vi "OxyChip Calibration Prompt.vi"(11 "Measurement Information In":T1={"Comments"="", "Directory Input"="", "Data file path"=path "C:/Data/EPR Data", "Scripting File"=path "C:/Data/Configuration Script.csv", "Save Data"=FALSE, "Tooth size (d11) [mm]"=0.0, "Tooth size (d12) [mm]"=0.0, "Tooth size (d21) [mm]"=0.0, "Tooth size (d22) [mm]"=0.0, "Dose of Tooth [Gy]"=0.0, "Safe Shutdown?"=FALSE, "Gases Available"=[], "Database Username"="", "Database Password"="", "Database Login URL"="", "Database Upload URL"="", "Database Success URL"="", "Database XML URL"="", "Database Resonator URL"="", "Session Number"=0, "Set #"=0, "Resonator Operator"="", "Session Type"="", "Tooth/Sample ID"="", "Volunteer ID"="", "Computer Operator"="", "Volunteer Type"="", "Site/Tooth Selection (T8,T9)"="", "Resonator"="", "Measurement Site"="", "Non-standard session?"=FALSE, "EPR DAQ Version"="", "Session Path"=path "C:/Data/EPR Data", "Chosen Applied State"="", "Chosen Initial State"="", "Time of Transition"="", "DAQ Mode"=enum."Engineering", "pO2/Scan [mmHg]"=[], "pO2/Set [mmHg]"=[], "Linewidth (HWHM)/Scan [Gauss]"=[], "Linewidth (HWHM)/Set [Gauss]"=[], "pO2 Conversion"="", "Dose Calibration Cluster"={"Dose Response"={"grand_mean"=0.0292016, "slope"=0.0188720543}, "Dose Correction"={"Sex"=1, "a0"=7.719669421, "a1"=-2.746550736, "a2"=-0.186490355, "a3"=0.041922063, "a4"=-0.849147359, "a5"=0.14330063, "a6"=0.019930219, "A_n"=40.0, "H_n"=10.12, "Dose Correction"=FALSE}, "Dose Reporting"={"Reporting is"=TRUE, "sd_threshold [AU]"=0.06, "sd_model [Gy]"=0.66, "dosimetric_threshold [Gy]"=2.0, "Add intrasession errors is"=FALSE, "Prior Radiation?"=FALSE}}, "OxyChip Slope"=0.0, "OxyChip Intercept"=0.0, "QA Mode"=enum."Select QA Mode", "QA Session?"=FALSE, "Sample Type"=enum."Empty Resonator", "Report pO2/Scan"=FALSE, "Skip End Session Save"=FALSE, "Number of sites"=enum."# Probes", "Recipient Name"="", "Sender Name"="", "Recipient Email"="", "Transition State History"=[], "pO2 Report Times"=[], "Temperature [C]"=0.0, "+Error pO2/Scan [mmHg]"=[], "-Error pO2/Scan [mmHg]"=[], "+Error pO2/Set [mmHg]"=[], "-Error pO2/Set [mmHg]"=[], "Oxy Phase Exclusion Tolerance [rad]"=0.0, "Oxy Center Exclusion Tolerance [%]"=0.0, "Oxy Exclude Unacceptable"=FALSE, "Oxy Unacceptable Estimate Flags"=[], "Save Session PPT"=FALSE, "Flagged Bad Sets"=[]} {"Oxy Center Exclusion Tolerance [%]" format="%#_9g"; "Oxy Phase Exclusion Tolerance [rad]" format="%#_9g"; "Temperature [C]" format="%#_9g"; "OxyChip Intercept" format="%#_9g"; "OxyChip Slope" format="%#_9g"; "Dose Calibration Cluster"."Dose Reporting"."dosimetric_threshold [Gy]" format="%#_9g"; "Dose Calibration Cluster"."Dose Reporting"."sd_model [Gy]" format="%#_9g"; "Dose Calibration Cluster"."Dose Reporting"."sd_threshold [AU]" format="%#_9g"; "Dose Calibration Cluster"."Dose Correction"."H_n" format="%#_9g"; "Dose Calibration Cluster"."Dose Correction"."A_n" format="%#_9g"; "Dose Calibration Cluster"."Dose Correction"."a6" format="%#.9g"; "Dose Calibration Cluster"."Dose Correction"."a5" format="%#.9g"; "Dose Calibration Cluster"."Dose Correction"."a4" format="%#.9g"; "Dose Calibration Cluster"."Dose Correction"."a3" format="%#.9g"; "Dose Calibration Cluster"."Dose Correction"."a2" format="%#.9g"; "Dose Calibration Cluster"."Dose Correction"."a1" format="%#.9g"; "Dose Calibration Cluster"."Dose Correction"."a0" format="%#.9g"; "Dose Calibration Cluster"."Dose Correction"."Sex" items=["Male"=1, "Female"=0]; "Dose Calibration Cluster"."Dose Response"."slope" format="%#_9g"; "Dose Calibration Cluster"."Dose Response"."grand_mean" format="%#_9g"}) -> (3 "Measurement Information Out":T1={"Comments"="", "Directory Input"="", "Data file path"=path "C:/Data/EPR Data", "Scripting File"=path "C:/Data/Configuration Script.csv", "Save Data"=FALSE, "Tooth size (d11) [mm]"=0.0, "Tooth size (d12) [mm]"=0.0, "Tooth size (d21) [mm]"=0.0, "Tooth size (d22) [mm]"=0.0, "Dose of Tooth [Gy]"=0.0, "Safe Shutdown?"=FALSE, "Gases Available"=[], "Database Username"="", "Database Password"="", "Database Login URL"="", "Database Upload URL"="", "Database Success URL"="", "Database XML URL"="", "Database Resonator URL"="", "Session Number"=0, "Set #"=0, "Resonator Operator"="", "Session Type"="", "Tooth/Sample ID"="", "Volunteer ID"="", "Computer Operator"="", "Volunteer Type"="", "Site/Tooth Selection (T8,T9)"="", "Resonator"="", "Measurement Site"="", "Non-standard session?"=FALSE, "EPR DAQ Version"="", "Session Path"=path "C:/Data/EPR Data", "Chosen Applied State"="", "Chosen Initial State"="", "Time of Transition"="", "DAQ Mode"=enum."Engineering", "pO2/Scan [mmHg]"=[], "pO2/Set [mmHg]"=[], "Linewidth (HWHM)/Scan [Gauss]"=[], "Linewidth (HWHM)/Set [Gauss]"=[], "pO2 Conversion"="", "Dose Calibration Cluster"={"Dose Response"={"grand_mean"=0.0292016, "slope"=0.0188720543}, "Dose Correction"={"Sex"=1, "a0"=7.719669421, "a1"=-2.746550736, "a2"=-0.186490355, "a3"=0.041922063, "a4"=-0.849147359, "a5"=0.14330063, "a6"=0.019930219, "A_n"=40.0, "H_n"=10.12, "Dose Correction"=FALSE}, "Dose Reporting"={"Reporting is"=TRUE, "sd_threshold [AU]"=0.06, "sd_model [Gy]"=0.66, "dosimetric_threshold [Gy]"=2.0, "Add intrasession errors is"=FALSE, "Prior Radiation?"=FALSE}}, "OxyChip Slope"=0.0, "OxyChip Intercept"=0.0, "QA Mode"=enum."Select QA Mode", "QA Session?"=FALSE, "Sample Type"=enum."Empty Resonator", "Report pO2/Scan"=FALSE, "Skip End Session Save"=FALSE, "Number of sites"=enum."# Probes", "Recipient Name"="", "Sender Name"="", "Recipient Email"="", "Transition State History"=[], "pO2 Report Times"=[], "Temperature [C]"=0.0, "+Error pO2/Scan [mmHg]"=[], "-Error pO2/Scan [mmHg]"=[], "+Error pO2/Set [mmHg]"=[], "-Error pO2/Set [mmHg]"=[], "Oxy Phase Exclusion Tolerance [rad]"=0.0, "Oxy Center Exclusion Tolerance [%]"=0.0, "Oxy Exclude Unacceptable"=FALSE, "Oxy Unacceptable Estimate Flags"=[], "Save Session PPT"=FALSE, "Flagged Bad Sets"=[]} {"Oxy Center Exclusion Tolerance [%]" format="%#_9g"; "Oxy Phase Exclusion Tolerance [rad]" format="%#_9g"; "Temperature [C]" format="%#_9g"; "OxyChip Intercept" format="%#_9g"; "OxyChip Slope" format="%#_9g"; "Dose Calibration Cluster"."Dose Reporting"."dosimetric_threshold [Gy]" format="%#_9g"; "Dose Calibration Cluster"."Dose Reporting"."sd_model [Gy]" format="%#_9g"; "Dose Calibration Cluster"."Dose Reporting"."sd_threshold [AU]" format="%#_9g"; "Dose Calibration Cluster"."Dose Correction"."H_n" format="%#_9g"; "Dose Calibration Cluster"."Dose Correction"."A_n" format="%#_9g"; "Dose Calibration Cluster"."Dose Correction"."a6" format="%#.9g"; "Dose Calibration Cluster"."Dose Correction"."a5" format="%#.9g"; "Dose Calibration Cluster"."Dose Correction"."a4" format="%#.9g"; "Dose Calibration Cluster"."Dose Correction"."a3" format="%#.9g"; "Dose Calibration Cluster"."Dose Correction"."a2" format="%#.9g"; "Dose Calibration Cluster"."Dose Correction"."a1" format="%#.9g"; "Dose Calibration Cluster"."Dose Correction"."a0" format="%#.9g"; "Dose Calibration Cluster"."Dose Correction"."Sex" items=["Male"=1, "Female"=0]; "Dose Calibration Cluster"."Dose Response"."slope" format="%#_9g"; "Dose Calibration Cluster"."Dose Response"."grand_mean" format="%#_9g"})   [LabVIEW 2016]
uses:
  Types/Measurement Information.ctl
  Analysis/Dose Calculation and Reporting/Dose Calculation Control.ctl
  Types/Sample Type.ctl
panel:
  in  "Report pO2 for each scan?":bool
  in  "Continue":bool
  in  "OxyChip Calibration Intercept":dbl
  in  "OxyChip Calibration Slope":dbl
  # "Please enter OxyChip Calibration Information"
  # "Session Information"
  # "Oximetric Data and Information"
  # "Email"
  # "Tooth Information"
  # "Database"
  # "Session Information"
  # "Oximetric Data and Information"
  # "Email"
  # "Tooth Information"
  # "Database"
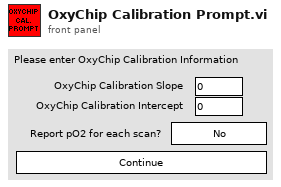
[diagram p1: front panel]
types:
  T1 = typedef "Measurement Information.ctl" = cluster{"Comments":string, "Directory Input":string, "Data file path":path, "Scripting File":path, "Save Data":bool, "Tooth size (d11) [mm]":dbl, "Tooth size (d12) [mm]":dbl, "Tooth size (d21) [mm]":dbl, "Tooth size (d22) [mm]":dbl, "Dose of Tooth [Gy]":dbl, "Safe Shutdown?":bool, "Gases Available":string[], "Database Username":string, "Database Password":string, "Database Login URL":string, "Database Upload URL":string, "Database Success URL":string, "Database XML URL":string, "Database Resonator URL":string, "Session Number":i32, "Set #":u32, "Resonator Operator":string, "Session Type":string, "Tooth/Sample ID":string, "Volunteer ID":string, "Computer Operator":string, "Volunteer Type":string, "Site/Tooth Selection (T8,T9)":string, "Resonator":string, "Measurement Site":string, "Non-standard session?":bool, "EPR DAQ Version":string, "Session Path":path, "Chosen Applied State":string, "Chosen Initial State":string, "Time of Transition":string, "DAQ Mode":enum16{"Engineering", "Dosimetry", "Oximetry"}, "pO2/Scan [mmHg]":dbl[][], "pO2/Set [mmHg]":dbl[][], "Linewidth (HWHM)/Scan [Gauss]":dbl[][], "Linewidth (HWHM)/Set [Gauss]":dbl[][], "pO2 Conversion":string, "Dose Calibration Cluster":T2, "OxyChip Slope":dbl, "OxyChip Intercept":dbl, "QA Mode":enum16{"Select QA Mode", "QA-Start/End", "QA-Mid", "QA-Weekly", "QA-Eng", "Check Calibration"}, "QA Session?":bool, "Sample Type":T3, "Report pO2/Scan":bool, "Skip End Session Save":bool, "Number of sites":enum16{"# Probes", "1", "2", "3", "4"}, "Recipient Name":string, "Sender Name":string, "Recipient Email":string, "Transition State History":string[], "pO2 Report Times":string[], "Temperature [C]":dbl, "+Error pO2/Scan [mmHg]":dbl[][], "-Error pO2/Scan [mmHg]":dbl[][], "+Error pO2/Set [mmHg]":dbl[][], "-Error pO2/Set [mmHg]":dbl[][], "Oxy Phase Exclusion Tolerance [rad]":dbl, "Oxy Center Exclusion Tolerance [%]":dbl, "Oxy Exclude Unacceptable":bool, "Oxy Unacceptable Estimate Flags":bool[], "Save Session PPT":bool, "Flagged Bad Sets":u32[]}
  T2 = typedef "Dose Calculation Control.ctl" = cluster{"Dose Response":cluster{"grand_mean":dbl, "slope":dbl}, "Dose Correction":cluster{"Sex":u16, "a0":dbl, "a1":dbl, "a2":dbl, "a3":dbl, "a4":dbl, "a5":dbl, "a6":dbl, "A_n":dbl, "H_n":dbl, "Dose Correction":bool}, "Dose Reporting":cluster{"Reporting is":bool, "sd_threshold [AU]":dbl, "sd_model [Gy]":dbl, "dosimetric_threshold [Gy]":dbl, "Add intrasession errors is":bool, "Prior Radiation?":bool}}
  T3 = typedef "Sample Type.ctl" = enum16{"Empty Resonator", "IRS", "BallZero", "Irradiated Tooth", "Non-irradiated Tooth", "OxyChip", "LiPc", "PDT", "India Ink"}
  T4 = enum8{"Enabled", "Disabled", "Disabled and Grayed Out"}
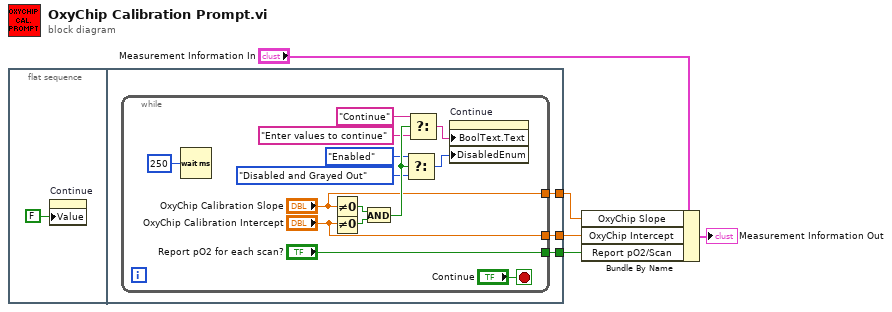
[diagram p0: block diagram]
diagram:
  n1 = flat-sequence {
    tunnel: [w9] -> w5
    tunnel: [w8] -> w4
    tunnel: [w7] -> w1
    frame #0 {
      n2 = property on="Continue" class="Bool (strict)"("Value"=FALSE ("Continue")) -> ()  [unwired: 2 in, 2 out]
    }
    frame #1 {
      n3 = while {
        tunnel: ["OxyChip Calibration Intercept"] -> w8
        tunnel: ["OxyChip Calibration Slope"] -> w9
        tunnel: ["Report pO2 for each scan?"] -> w7
        stop <- "Continue" stop-if-true
        n4 = Wait (ms)(milliseconds to wait=u32 250) -> ()  [unwired: 1 out]
        n5 = Not Equal To 0?(x="OxyChip Calibration Slope") -> (x != 0?=w22:bool)
        n6 = Not Equal To 0?(x="OxyChip Calibration Intercept") -> (x != 0?=w23:bool)
        n7 = And(x=w22, y=w23) -> (x .and. y?=w21:bool)
        n8 = Select(t=T4."Enabled" ("Disabled"), s=w21, f=T4."Disabled and Grayed Out" ("Disabled")) -> (s? t:f=w18:T4)
        n9 = Select(t="Continue" ("Boolean Text.Text"), s=w21, f="Enter values to continue" ("Boolean Text.Text")) -> (s? t:f=w15:string)
        n10 = property on="Continue" class="Bool (strict)"("BoolText.Text"=w15, "DisabledEnum"=w18) -> ()  [unwired: 2 in, 2 out]
      }
    }
  }
  n11 = Bundle By Name(cluster="Measurement Information In", "OxyChip Slope"=w5, "OxyChip Intercept"=w4, "Report pO2/Scan"=w1) -> (→"Measurement Information Out":T1)
